vi "m1m3_issueCommand_RunMirrorForceProfile.vi"(8 "error in (no error)":errorcluster, 11 "command_RunMirrorForceProfile_Ctl":T1={"XForce[1000]"=array[1000 elements], "YForce[1000]"=array[1000 elements], "ZForce[1000]"=array[1000 elements], "XMoment[1000]"=array[1000 elements], "YMoment[1000]"=array[1000 elements], "ZMoment[1000]"=array[1000 elements]}) -> (0 "error out":errorcluster, 2 "function return":i32, 3 "command_RunMirrorForceProfile_Ctl out":T1)   [LabVIEW 2016, in "SALLV_m1m3.lvlib"]
doc: "int m1m3_shm_issueCommand_RunMirrorForceProfileLV(m1m3_command_RunMirrorForceProfileLV *command_RunMirrorForceProfile_Ctl );"
uses:
  SALLV_m1m3.lvlib
  DataTypes/command_RunMirrorForceProfile.ctl
  SALLV_m1m3.so
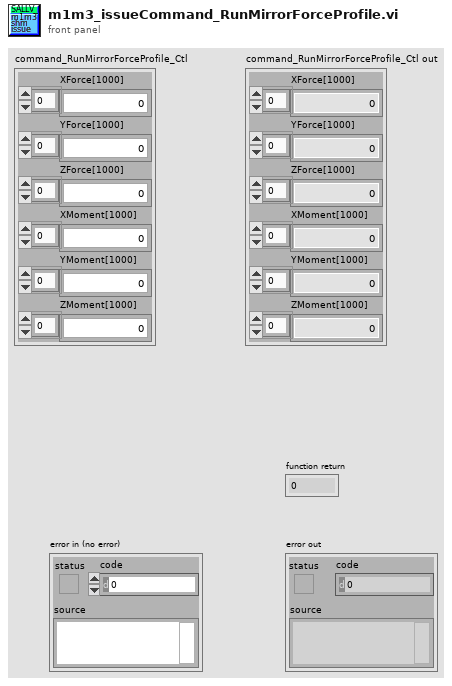
[diagram p1: front panel]
types:
  T1 = typedef "SALLV_m1m3.lvlib/command_RunMirrorForceProfile.ctl" = cluster{"XForce[1000]":sgl[], "YForce[1000]":sgl[], "ZForce[1000]":sgl[], "XMoment[1000]":sgl[], "YMoment[1000]":sgl[], "ZMoment[1000]":sgl[]}
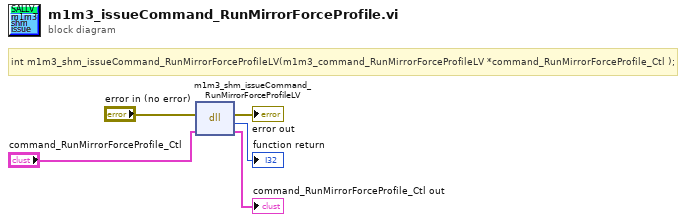
[diagram p0: block diagram]
diagram:
  # "int m1m3_shm_issueCommand_RunMirrorForceProfileLV(m1m3_command_RunMirrorForceProfileLV *command_RunMirrorForceProfile_Ctl );"
  n1 = dll-call lib="opt/CODE/SALLV_m1m3/SALLV_m1m3.*" fn="m1m3_shm_issueCommand_RunMirrorForceProfileLV"(error in="error in (no error)", "command_RunMirrorForceProfile_Ctl"="command_RunMirrorForceProfile_Ctl") -> (error out=→"error out":errorcluster, →"function return":i32, "command_RunMirrorForceProfile_Ctl"=→"command_RunMirrorForceProfile_Ctl out":T1)  [unwired: 2 in, 1 out]
